vi "Attach Observer.vi"(10 "Observer(s)":refnum<class "Send.lvclass">, 11 "Parallel Process in":refnum<class "Parallel Process.lvclass">) -> (3 "Parallel Process out":refnum<class "Parallel Process.lvclass">)   [LabVIEW 2011, in "Messenging.lvlib" / "Parallel Process.lvclass"]
uses:
  Parallel Process.lvclass
  Interprocess Messenger/Send/Send.lvclass
  Parallel Process.lvclass/Parallel Process.ctl
  Interprocess Messenger/Messenger (Parent)/MGR.lvclass
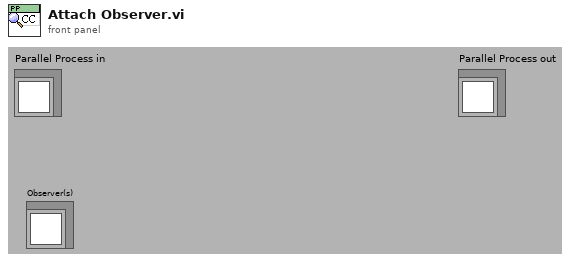
[diagram p1: front panel]
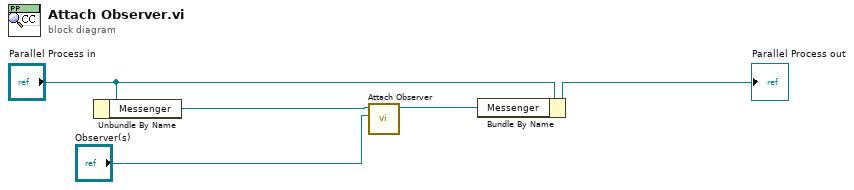
[diagram p0: block diagram]
diagram:
  n1 = Unbundle By Name("Parallel Process in") -> ("Messenger"=w3:refnum<class "MGR.lvclass">)
  n2 = call "Attach Observer.vi"("Observer(s)"="Observer(s)", "MGR.lvclass in"=w3) -> ("MGR.lvclass out"=w2:refnum<class "MGR.lvclass">)  [unwired: 1 in, 8 out]
  n3 = Bundle By Name(cluster="Parallel Process in", "Messenger"=w2) -> (→"Parallel Process out":refnum<class "Parallel Process.lvclass">)
